vi "Get IController .NET.vi"(11 "Tool Tip Text in":refnum<class "Tool Tip Text.lvclass">) -> (2 "IController":refnum<k24>, 3 "Tool Tip Text out":refnum<class "Tool Tip Text.lvclass">)   [LabVIEW 2023, in "SourceGrid.lvlib" / "Tool Tip Text.lvclass"]
uses:
  Tool Tip Text.lvclass
  D:/git/Sourcegrid-LabVIEW/dll/SourceGrid.dll
  dll/SourceGrid.dll
  Tool Tip Text.lvclass/Tool Tip Text.ctl
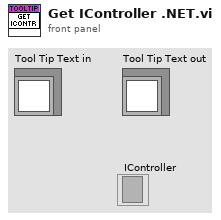
[diagram p1: front panel]
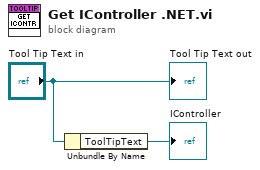
[diagram p0: block diagram]
diagram:
  n1 = Unbundle By Name("Tool Tip Text in") -> ("ToolTipText"=→"IController":refnum<k24>)
  "Tool Tip Text out" <- "Tool Tip Text in"
